vi "GetText.vi"(8 "error in":errorcluster, 11 "Modbus Slave editor node in":refnum<class "Modbus Module editor node.lvclass">) -> (0 "error out":errorcluster, 1 "additional text":string, 2 "text":string, 3 "Modbus Slave editor node out":refnum<class "Modbus Module editor node.lvclass">, 4 "glyph":string)   [LabVIEW 2013, in "Modbus Module editor node.lvclass"]
doc: "Platypus Framework 1.0.1.65\nNI Systems Engineering - National Instruments"
uses:
  Modbus Module editor node.lvclass
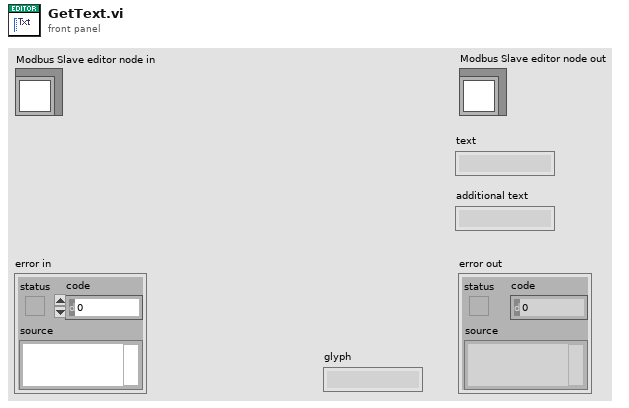
[diagram p1: front panel]
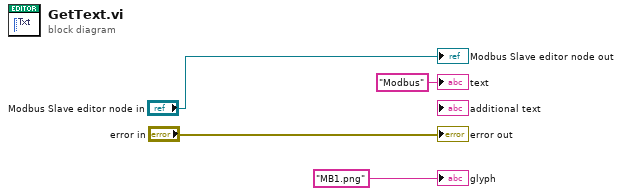
[diagram p0: block diagram]
diagram:
  "error out" <- "error in"
  "Modbus Slave editor node out" <- "Modbus Slave editor node in"
  "text" <- "Modbus" ("text")
  "glyph" <- "MB1.png" ("glyph")
